vi "Run Test (VIRefnum Scalar).vi"(4 "timeout (2000 ms)":i32=2000, 5 "Test Report":refnum<class "Test Report.lvclass">, 6 "Verbose":bool, 7 "Report Path":path, 8 "error in":errorcluster, 9 "Inspect Recursively (T)":bool=TRUE, 10 "VI Refnum":refnum<vi>, 11 "Interactive (T)":bool=TRUE) -> (0 "error out":errorcluster, 3 "Test Results":refnum<class "Test Result.lvclass">)   [LabVIEW 2020, in "Caraya.lvlib"]
doc: "\"Run Tests\" from a VI reference:\n- Dynamically discovers Caraya unit tests from a VI reference and runs them\n- Outputs results in a UI ans/or Test Report (J-Unit or text)\n\n(Not compatible with RT targets or RunTime Engine)"
uses:
  Caraya.lvlib
  classes/Test Report/Test Report.lvclass
  classes/Test Result/Test Result.lvclass
  classes/Test Runner.Folder/Test Runner.Folder.lvclass
  C:/projects/caraya/src/classes/Test Runner/Test Runner.lvclass
  classes/Test Runner/Test Runner.lvclass
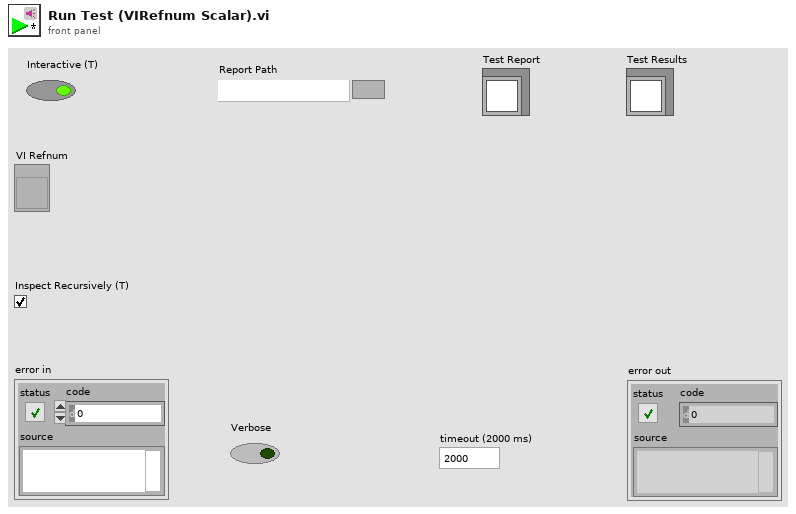
[diagram p1: front panel]
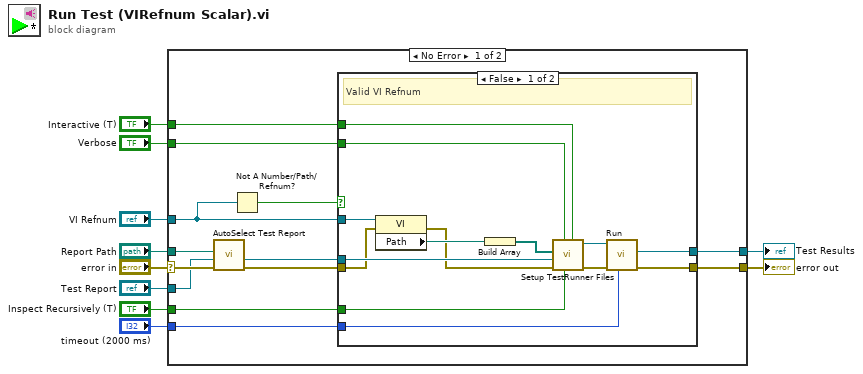
[diagram p0: block diagram]
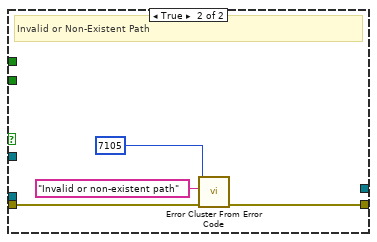
[diagram p2: hidden frame]
diagram:
  n1 = case shown="No Error" "error in" {
    selector: "error in" -> [w20 w42]
    tunnel: [w23 w42] -> w10
    tunnel: "Verbose" -> [w22 _]
    tunnel: "Interactive (T)" -> [w21 _]
    tunnel: "Test Report" -> [w17 _]
    tunnel: "VI Refnum" -> [w14 _]
    tunnel: "Report Path" -> [w19 _]
    tunnel: "Inspect Recursively (T)" -> [w15 _]
    tunnel: "timeout (2000 ms)" -> [w12 _]
    tunnel: [w11 _] -> w1
    frame No Error {
      n2 = call "AutoSelect Test Report.vi"("error in (no error)"=w20, "Test Report in"=w17, "Report Path"=w19) -> ("error out"=w18:errorcluster, "Test Report out"=w16:refnum<class "Test Report.lvclass">)  [unwired: 7 in]
      n3 = Not A Number/Path/Refnum?(number/path/refnum=w14) -> (NaN/Path/Refnum?=w13:bool)
      n4 = case shown="False" w13 {
        tunnel: [w37 w40] -> w23
        tunnel: w22 -> [w35 _]
        tunnel: w21 -> [w34 _]
        tunnel: w18 -> [w27 w41]
        tunnel: w16 -> [w32 _]
        tunnel: w15 -> [w31 _]
        tunnel: w14 -> [w29 _]
        tunnel: w12 -> [w25 _]
        tunnel: [w24 _] -> w11
        frame False {
          # "Valid VI Refnum"
          n5 = property class="VI"(reference=w29, error in=w27) -> (error out=w26:errorcluster, "Path"=w28:path)  [unwired: 1 out]
          n6 = Build Array(w28) -> (w30:path[])
          n7 = call "Setup TestRunner Files.vi"("Interactive (T)"=w34, "Inspect Recursively (T)"=w31, "Verbose (F)"=w35, "error in (no error)"=w26, "Test Report"=w32, "Paths"=w30) -> ("error out"=w36:errorcluster, "Test Runner.Folder out"=w33:refnum<class "Test Runner.Folder.lvclass">)  [unwired: 4 in]
          n8 = call "Run.vi"("timeout"=w25, "error in (no error)"=w36, "Test Runner in"=w33) -> ("error out"=w37:errorcluster, "Test Suite Results"=w24:refnum<class "Test Result.lvclass">)  [unwired: 6 in, 1 out]
        }
        frame True {
          # "Invalid or Non-Existent Path"
          n9 = call <vilib>:"Error Cluster From Error Code.vi"("error in (no error)"=w41, "error message (\"\")"="Invalid or non-existent path" ("error message (\"\")"), "error code (0)"=7105 ("code")) -> ("error out"=w40:errorcluster)  [unwired: 6 in]
        }
      }
    }
    frame Error {
    }
  }
  "error out" <- w10
  "Test Results" <- w1
